vi "create filepath list.vi"(1 "regular expression":string, 2 "folder path (not file)":path) -> (0 "Array":path[](array[path]))   [LabVIEW 2024]
uses:
  <vilib>/regexp/Match Regular Expression.xnode
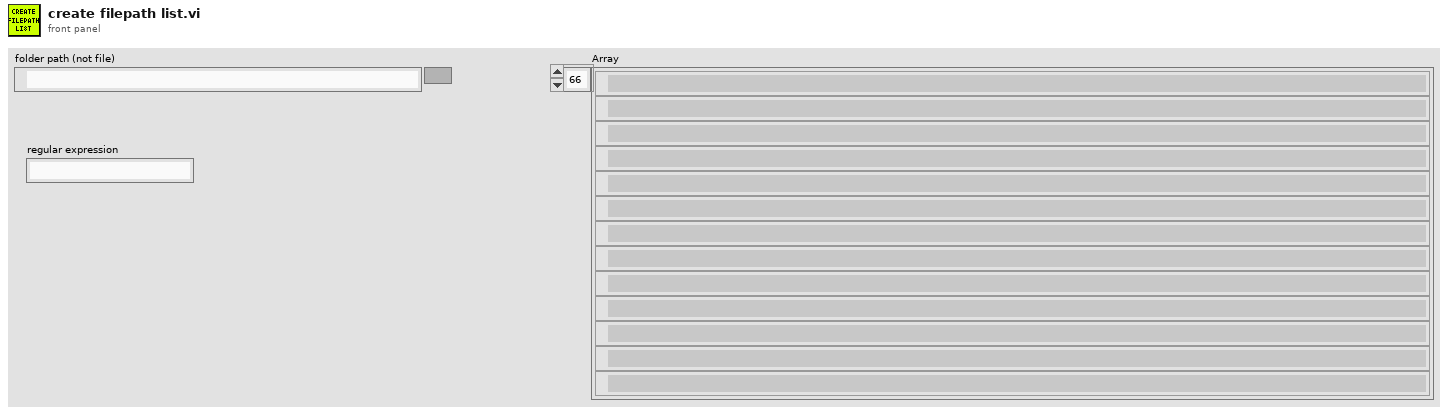
[diagram p1: front panel]
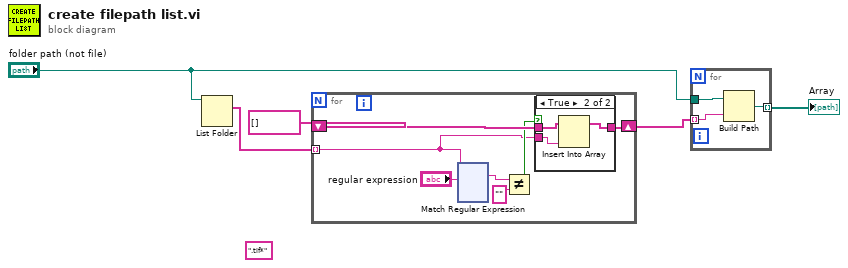
[diagram p0: block diagram]
diagram:
  (unwired) ".tif*" ("regular expression")
  n1 = List Folder(path="folder path (not file)") -> (filenames=w3:string[])  [unwired: 3 in, 3 out]
  n2 = for {
    tunnel: w3 -> [w7] mode=indexing
    shift-right: [w9] -> w2
    shift-left: string[] [] -> [w10]
    n3 = xnode "Match Regular Expression"("input string"=w7, "regular expression"="regular expression") -> ("whole match"=w11:string)  [unwired: 4 in, 4 out]
    n4 = Not Equal?(x=w11, y="") -> (x != y?=w8:bool)
    n5 = case shown="True" w8 {
      tunnel: w10 -> [w13 w16]
      tunnel: [w13 w15] -> w9
      tunnel: w7 -> [_ w14]
      frame False {
      }
      frame True {
        n6 = Insert Into Array(array=w16, new element=w14) -> (w15:string[])  [unwired: 1 in]
      }
    }
  }
  n7 = for {
    tunnel: w2 -> [w136] mode=indexing
    tunnel: "folder path (not file)" -> [w135]
    tunnel: [w134] -> w5 mode=indexing
    n8 = Build Path(base path=w135, name or relative path=w136) -> (appended path=w134:path)
  }
  "Array" <- w5
